vi "Write Data Ref.vi"(8 "error in (no error)":errorcluster, 10 "Data Table Ref":T1, 11 "Simulated VeriStand Engine in":refnum<class "Simulated VeriStand Engine.lvclass">) -> (0 "error out":errorcluster, 3 "Simulated VeriStand Engine out":refnum<class "Simulated VeriStand Engine.lvclass">)   [LabVIEW 2016, in "Simulated VeriStand Engine.lvclass"]
uses:
  Simulated VeriStand Engine.lvclass
  <vilib>/NI Veristand/Custom Device API/Data Table Ref.ctl
  Simulated VeriStand Engine.lvclass/Simulated VeriStand Engine.ctl
  <vilib>/NI Veristand/Custom Device API/Global Data Refs.vi
  <vilib>/NI Veristand/Custom Device API/Custom Device API.lvlib
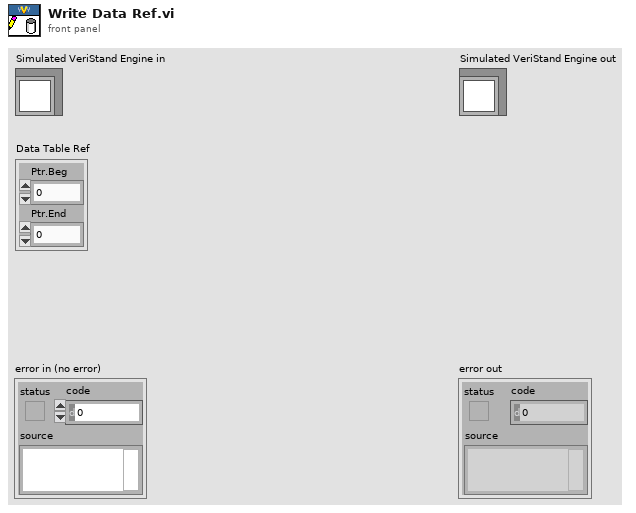
[diagram p1: front panel]
types:
  T1 = typedef "Custom Device API.lvlib/Data Table Ref.ctl" = cluster{"Ptr.Beg":u64, "Ptr.End":u64}
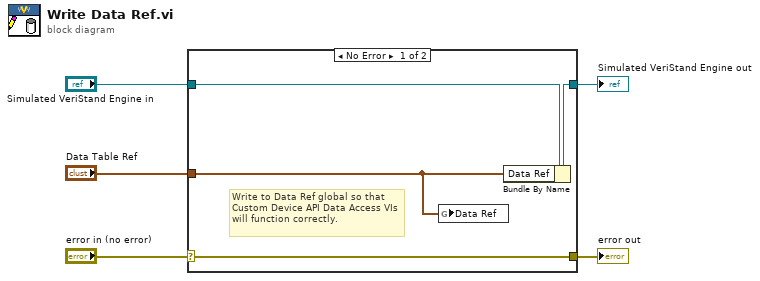
[diagram p0: block diagram]
diagram:
  n1 = case shown="No Error" "error in (no error)" {
    selector: "error in (no error)" -> [w9 w10]
    tunnel: [w9 w10] -> w4
    tunnel: [w7 w11] -> w2
    tunnel: "Simulated VeriStand Engine in" -> [w8 w11]
    tunnel: "Data Table Ref" -> [w6 _]
    frame No Error {
      # "Write to Data Ref global so that Custom Device API Data Access VIs will function correctly."
      n2 = global write "Global Data Refs.vi" "Data Ref"(w6) -> ()
      n3 = Bundle By Name(cluster=w8, "Data Ref"=w6) -> (w7:refnum<class "Simulated VeriStand Engine.lvclass">)
    }
    frame Error {
    }
  }
  "error out" <- w4
  "Simulated VeriStand Engine out" <- w2
